vi "check-state-switch.vi"() -> ()   [LabVIEW 2021]
panel:
  in  "Con_State":u8(ring) items=["Idle"=0, "Busy"=1, "Wait4srcON"=2, "Ready"=3, "Forming"=5, "Feeding"=6, "Error"=9, "Wait4srcOFF"=10, "ISRC mode"=11, "VSRC mode"=12]
  in  "mode":dbl
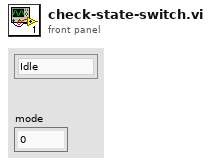
[diagram p1: front panel]
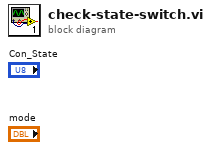
[diagram p0: block diagram]
diagram:
